vi "Internal Accelerometer.vi"() -> ()   [LabVIEW 2025]
doc: "This example shows how to use the internal accelerometer built into the roboRIO. It reads X, Y, and Z axis acceleration.\n\nThis example expects a USB cable connected from your development PC to the Type B USB Jack (next to the power input) on the roboRIO."
uses:
  <vilib>/Rock Robotics/WPI/Accelerometer/WPI_AccelerometerRange.ctl
  <vilib>/Rock Robotics/WPI/Accelerometer/InternalAccelerometer/WPI_AccelerometerInternalOpen.vi
panel:
  in  "Accel Range":T1
  out "Z Acceleration":dbl
  out "Y Acceleration":dbl
  out "X Acceleration":dbl
  out "error out":errorcluster
  in  "stop":bool
  # "Set this input before running."
  # "Output information"
  # "This uses the internal accelerometer built into the roboRIO.  No wiring is necessary."
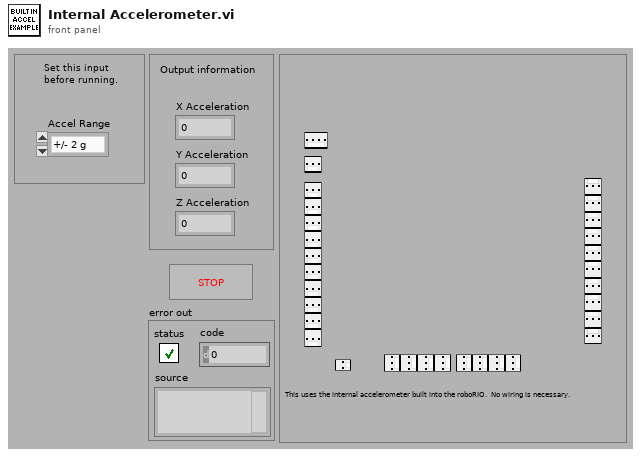
[diagram p1: front panel]
types:
  T1 = typedef "WPI_AccelerometerRange.ctl" = enum16{"+/- 2 g", "+/- 4 g", "+/- 8 g"}
  T2 = typedef "WPI_AccelerometerDevRef.ctl" = cluster{"DevStatus":errorcluster, "Scaling":T3, "Analog Channels":T4, "I2C Bus":T6, "SPI Bus":T7, "Accel Range":T8, "ADXL Axes":T9, "Handle":i32, "Device Address":u8, "Accel Type":enum16{"Analog", "ADXL345 I2C", "ADXL345 SPI", "Internal", "ADXL362 SPI"}}
  T3 = typedef "WPI_AccelerometerScaling.ctl" = cluster{"Gain (VoltsPerG)":dbl, "Center Voltage":dbl}
  T4 = typedef "WPI_AccelerometerAnalogChannels.ctl" = cluster{"X-Axis":T5, "Y-Axis":T5, "Z-Axis":T5}
  T5 = typedef "FPGA_AIChannel.ctl" = enum8{"AI 0", "AI 1", "AI 2", "AI 3", "AI MXP 0", "AI MXP 1", "AI MXP 2", "AI MXP 3", "Invalid"}
  T6 = typedef "i2c_bus.ctl" = enum16{"I2C On-Board", "I2C MXP", "Invalid"}
  T7 = typedef "spi_bus.ctl" = enum16{"SPI On-Board, CS0", "SPI On-Board, CS1", "SPI On-Board, CS2", "SPI On-Board, CS3", "SPI MXP", "Invalid"}
  T8 = typedef "ADXL345 Range.ctl" = u8
  T9 = typedef "WPI_AccelerometerADXL345 Axes.ctl" = cluster{"X-Axis":bool, "Y-Axis":bool, "Z-Axis":bool}
  T10 = cluster{"X-Axis":dbl, "Y-Axis":dbl, "Z-Axis":dbl}
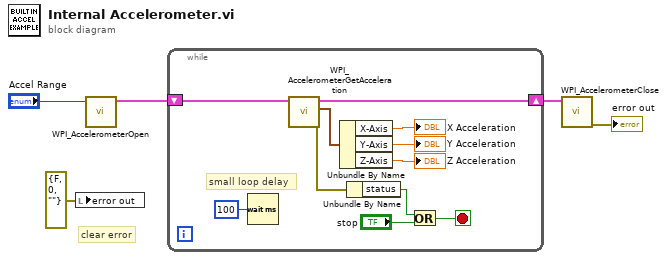
[diagram p0: block diagram]
diagram:
  # "clear error"
  n1 = local write "error out"(errorcluster {"status"=FALSE, "code"=0, "source"=""} ("error out")) -> ()
  n2 = call-poly <vilib>:"WPI_AccelerometerOpen.vi"("Accel Range"="Accel Range") -> ("AccelerometerDevRef"=w5:T2)  [unwired: 9 in, 1 out]
  n3 = while {
    shift-right: [w12] -> w3
    shift-left: w5 -> [w10]
    stop <- w11 stop-if-true
    # "small loop delay"
    n4 = Wait (ms)(milliseconds to wait=u32 100) -> ()  [unwired: 1 out]
    n5 = call <vilib>:"WPI_AccelerometerGetAcceleration.vi"("AccelerometerDevRef"=w10) -> ("error out"=w9:errorcluster, "Accelerations"=w13:T10, "AccelerometerDevRef"=w12:T2)  [unwired: 8 in]
    n6 = Unbundle By Name(w13) -> ("X-Axis"=→"X Acceleration":dbl, "Y-Axis"=→"Y Acceleration":dbl, "Z-Axis"=→"Z Acceleration":dbl)
    n7 = Unbundle By Name(w9) -> ("status"=w16:bool)
    n8 = Or(x=w16, y="stop") -> (x .or. y?=w11:bool)
  }
  n9 = call <vilib>:"WPI_AccelerometerClose.vi"("AccelerometerDevRef"=w3) -> ("error out"=→"error out":errorcluster)  [unwired: 10 in]
